vi "NeuronID_UDP_send_v001.vi"(2 "error in (no error)":errorcluster, 3 "Neuron ID":dbl(slide) scale=0.0..10.0, 4 "Address selector":i32[](array[numeric]), 5 "UDP Network Connection in":refnum<k16>) -> (0 "error out":errorcluster, 1 "UDP Network Connection out":refnum<k16>)   [LabVIEW 2019]
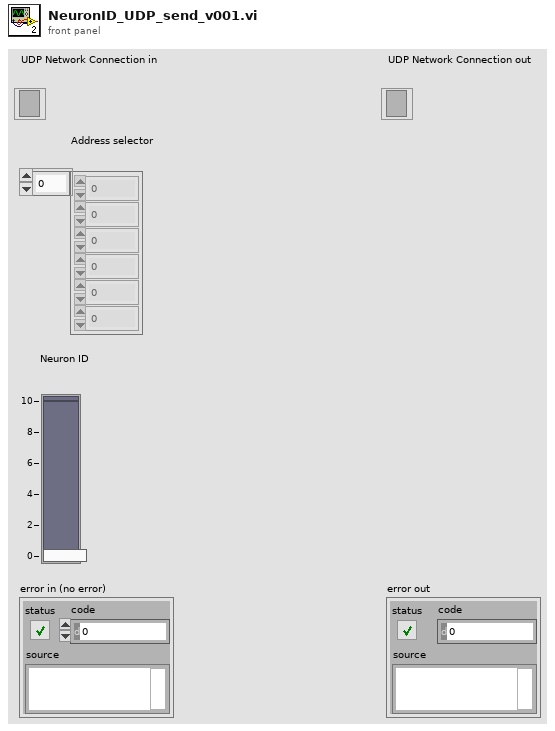
[diagram p1: front panel]
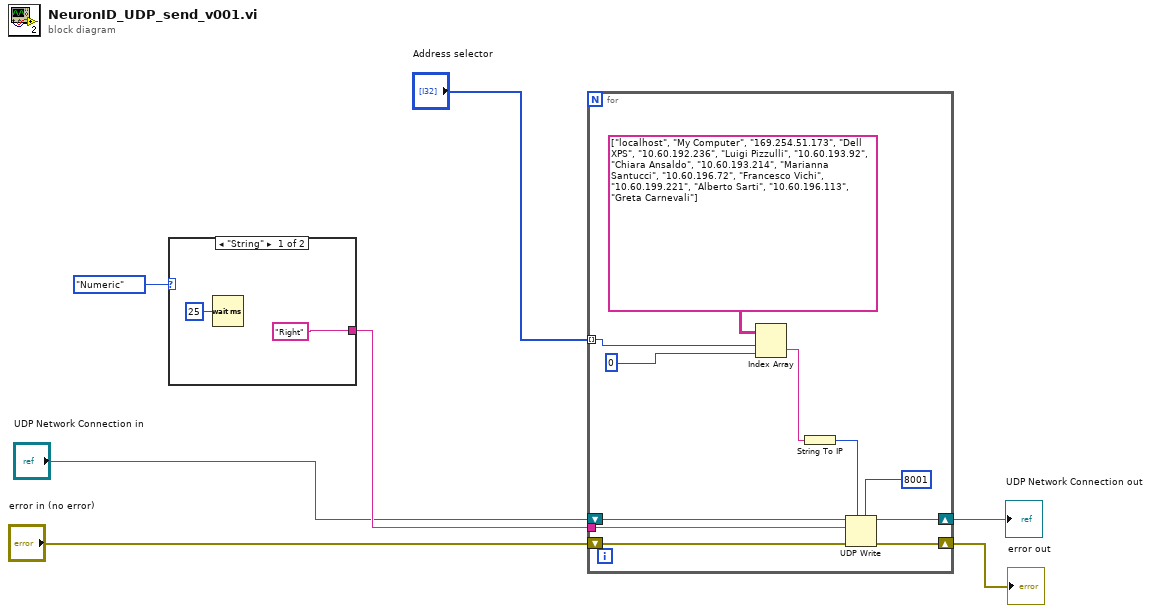
[diagram p0: block diagram]
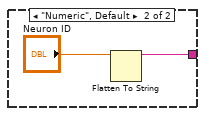
[diagram p2: hidden frame]
diagram:
  n1 = case shown="\"String\"" enum16{"String", "Numeric"}."Numeric" ("Data to send") {
    tunnel: ["Right" ("Message") w10] -> w6
    frame "String" {
      n2 = Wait (ms)(milliseconds to wait=u32 25) -> ()  [unwired: 1 out]
    }
    frame "Numeric", Default {
      n3 = Flatten To String(anything="Neuron ID") -> (data string=w10:string)  [unwired: 3 in, 2 out]
    }
  }
  n4 = for {
    tunnel: w6 -> [w16]
    shift-right: [w21] -> w2
    shift-left: "error in (no error)" -> [w22]
    shift-right: [w19] -> w4
    shift-left: "UDP Network Connection in" -> [w20]
    tunnel: "Address selector" -> [w12] mode=indexing
    n5 = Index Array(array=string[][] [["localhost", "My Computer"], ["169.254.51.173", "Dell XPS"], ["10.60.192.236", "Luigi Pizzulli"], ["10.60.193.92", "Chiara Ansaldo"], ["10.60.193.214", "Marianna Santucci"], ["10.60.196.72", "Francesco Vichi"], ["10.60.199.221", "Alberto Sarti"], ["10.60.196.113", "Greta Carnevali"]] ("Address list"), index (row)=w12, index (col)=0 ("disabled index (col)")) -> (element=w13:string)
    n6 = String To IP(1:w13) -> (0:w17:u32)
    n7 = UDP Write(address=w17, port or service name=u16 8001, connection ID=w20, data in=w16, 8:w22) -> (error out=w21:errorcluster, 3:w19:refnum<k16>)  [unwired: 1 in]
  }
  "UDP Network Connection out" <- w4
  "error out" <- w2
